vi "GEA3 Set EMV Exact Position.vi"(8 "error in (no error)":errorcluster, 9 "EMV Position":i16, 10 "Disable EMV GEA Flow":bool, 11 ".NET Refnum in":refnum<k24>) -> (0 "error out":errorcluster, 1 "Initial Mix Valve Position":u16, 2 "Final Mix Valve Position":u16, 3 ".NET Refnum out":refnum<k24>)   [LabVIEW 2019]
uses:
  C:/TechnologyLab/NI-2010/Drivers/GEA3 Toolkit/GEA3 DLL Source/GeaCommunication.dll
  GEA3 DLL Source/GeaCommunication.dll
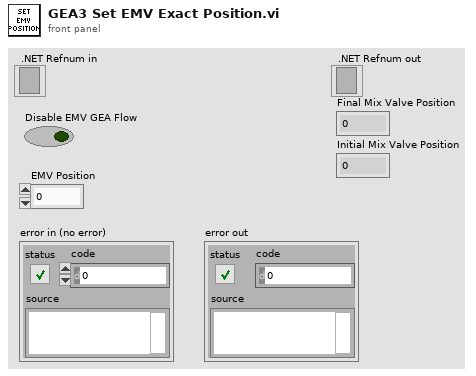
[diagram p1: front panel]
types:
  T1 = typedef "GEA2_Toolkit.lvlib/Source_Destination.ctl" = cluster{"Source":u8, "Destination":u8}
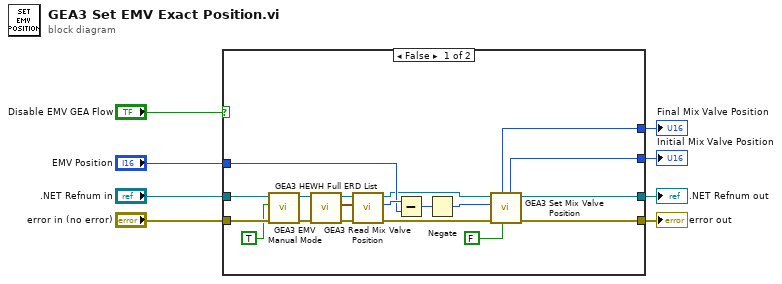
[diagram p0: block diagram]
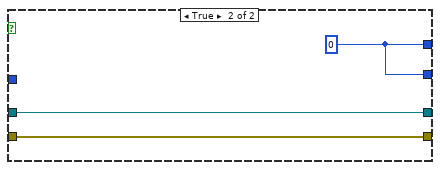
[diagram p2: hidden frame]
diagram:
  n1 = case shown="False" "Disable EMV GEA Flow" {
    tunnel: "error in (no error)" -> [w27 w30]
    tunnel: [w18 w30] -> w7
    tunnel: ".NET Refnum in" -> [w25 w29]
    tunnel: "EMV Position" -> [w16 _]
    tunnel: [w11 w29] -> w3
    tunnel: [w10 w28] -> w2
    tunnel: [w9 w28] -> w1
    frame False {
      n2 = call "GEA3 EMV Manual Mode.vi"("error in (no error)"=w27, "Manual Mode?"=TRUE, ".NET Refnum in"=w25) -> ("error out"=w21:errorcluster, "GEA2 Reference Out"=w20:refnum<k24>)  [unwired: 7 in]
      n3 = call "GEA3 HEWH Full ERD List.vi"("error in (no error)"=w21, "GEA2 Reference In"=w20) -> ("error out"=w22:errorcluster, "GEA Inputs"=w24:T1, "GEA2 Reference Out"=w23:refnum<k24>)  [unwired: 5 in, 2 out]
      n4 = call "GEA3 Read Mix Valve Position.vi"("error in (no error)"=w22, "GEA Inputs"=w24, ".NET Refnum in"=w23) -> ("error out"=w12:errorcluster, "Mix Valve Position"=w17:i16, ".NET Refnum out"=w14:refnum<k24>)  [unwired: 6 in]
      n5 = Subtract(x=w17, y=w16) -> (x-y=w15:i16)
      n6 = Negate(x=w15) -> (-x=w13:i16)
      n7 = call "GEA3 Set Mix Valve Position.vi"("Disable Check"=FALSE, "error in (no error)"=w12, "MIX VALVE STEP OFFSET (0x400A)"=w13, ".NET Refnum in"=w14) -> ("error out"=w18:errorcluster, ".NET Refnum out"=w11:refnum<k24>, "Initial Mix Valve Position"=w9:u16, "Final Mix Valve Position"=w10:u16)  [unwired: 2 in, 2 out]
    }
    frame True {
      w28 = u16 0 ("Final Mix Valve Position")
    }
  }
  "error out" <- w7
  ".NET Refnum out" <- w3
  "Final Mix Valve Position" <- w2
  "Initial Mix Valve Position" <- w1
